vi "log_record_file.vi"(11 "st_LogEvent":string) -> (0 "error out":errorcluster)   [LabVIEW 2026]
doc: "This subVI obtain time stamp from system to creates and write on log file the event"
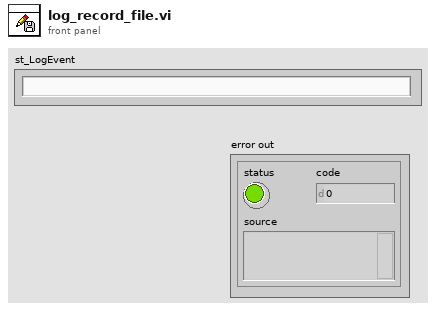
[diagram p1: front panel]
types:
  T1 = enum16{"open", "replace", "create", "open or create", "replace or create", "replace or create with confirmation"}
  T2 = cluster{"second":string, "minute":string, "hour":string, "day":string, "month":string, "year":string}
  T3 = typedef "LVDateTimeRec.ctl" = cluster{"fractional second":dbl, "second":i32, "minute":i32, "hour":i32, "day of month":i32, "month":i32, "year":i32, "day of week":i32, "day of year":i32, "DST":i32}
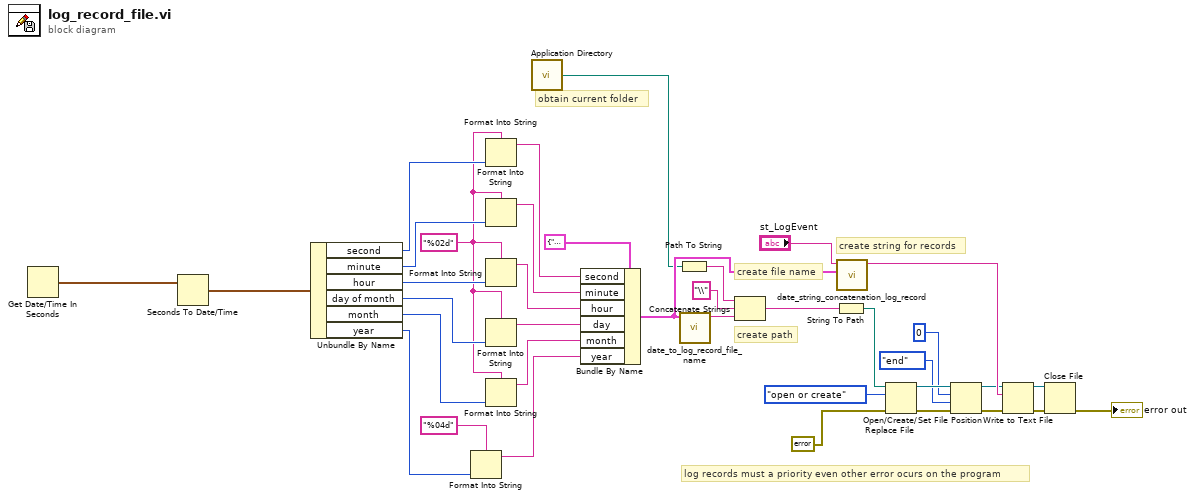
[diagram p0: block diagram]
diagram:
  w8 = "%02d"
  # "log records must a priority even other error ocurs on the program"
  # "create path"
  # "obtain current folder"
  # "create string for records"
  # "create file name"
  n1 = Get Date/Time In Seconds() -> (seconds since 1Jan1904=w34:timestamp)
  n2 = Seconds To Date/Time(time stamp (now)=w34) -> (date time rec=w35:T3)  [unwired: 1 in]
  n3 = Unbundle By Name(w35) -> ("second"=w33:i32, "minute"=w32:i32, "hour"=w31:i32, "day of month"=w30:i32, "month"=w29:i32, "year"=w28:i32)
  n4 = Format Into String(format string="%04d", w28) -> (resulting string=w26:string)  [unwired: 2 in, 1 out]
  n5 = Format Into String(format string=w8, w33) -> (resulting string=w25:string)  [unwired: 2 in, 1 out]
  n6 = Format Into String(format string=w8, w32) -> (resulting string=w24:string)  [unwired: 2 in, 1 out]
  n7 = Format Into String(format string=w8, w31) -> (resulting string=w23:string)  [unwired: 2 in, 1 out]
  n8 = Format Into String(format string=w8, w30) -> (resulting string=w22:string)  [unwired: 2 in, 1 out]
  n9 = Format Into String(format string=w8, w29) -> (resulting string=w21:string)  [unwired: 2 in, 1 out]
  n10 = call <vilib>:"Application Directory.vi"() -> ("Application Directory"=w16:path)
  n11 = Bundle By Name(cluster=T2 {"second"="", "minute"="", "hour"="", "day"="", "month"="", "year"=""}, "second"=w25, "minute"=w24, "hour"=w23, "day"=w22, "month"=w21, "year"=w26) -> (w19:T2)
  n12 = Path To String(path=w16) -> (string=w14:string)
  n13 = call "date_to_log_record_file_name.vi"("Cluster"=w19) -> ("st_logfilename"=w13:string)  [unwired: 10 in]
  n14 = Concatenate Strings(w14, "\\", w13) -> (w12:string)
  n15 = String To Path(string=w12) -> (path=w11:path)
  n16 = call "date_string_concatenation_log_record.vi"("Cluster"=w19, "st_LogEvent"="st_LogEvent") -> ("st_logrecord"=w10:string)  [unwired: 9 in]
  n17 = Open/Create/Replace File(file path (use dialog)=w11, error in=errorcluster {"status"=FALSE, "code"=0, "source"=""}, operation (0:open)=T1."open or create") -> (refnum out=w6:refnum<file>, error out=w5:errorcluster)  [unwired: 3 in, 1 out]
  n18 = Set File Position(offset (in bytes) (0)=i64 0, refnum=w6, from (0:start)=enum16{"start", "end", "current"}."end", error in=w5) -> (refnum out=w1:refnum<file>, error out=w4:errorcluster)
  n19 = Write to Text File(file (use dialog)=w1, text=w10, error in=w4) -> (refnum out=w17:refnum<file>, error out=w18:errorcluster)  [unwired: 1 in, 1 out]
  n20 = Close File(refnum=w17, error in=w18) -> (error out=→"error out":errorcluster)  [unwired: 1 out]
